vi "Example Websockets Client-Server.vi"() -> ()   [LabVIEW 2013]
uses:
  <vilib>/LabVIEW Open Source Project/Connection/Connection/Connection.lvclass
  MQTT_Websockets/Connection/WebsocketsConnection.lvclass
panel:
  out "server connected":bool
  out "client connected":bool
  out "Comm OK":bool
  out "value":dbl
  out "listener error":errorcluster
  out "client session error":errorcluster
  out "server session error":errorcluster
  out "Bytes":u8[](array[numeric]) format="%08b"
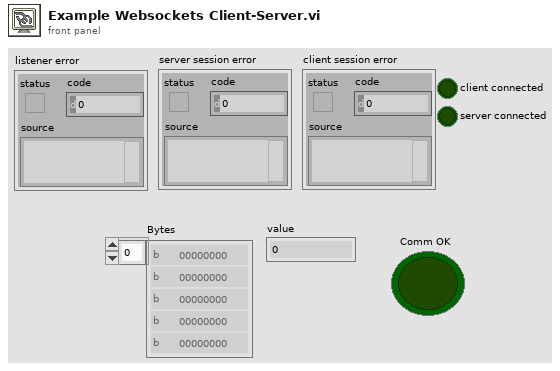
[diagram p1: front panel]
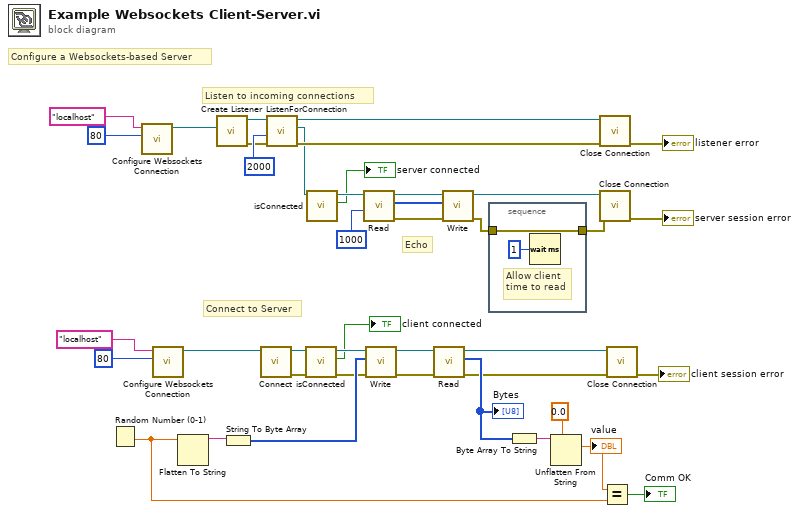
[diagram p0: block diagram]
diagram:
  # "Connect to Server"
  # "Echo"
  # "Listen to incoming connections"
  # "Configure a Websockets-based Server"
  n1 = Random Number (0-1)() -> (number: 0 to 1=w18:dbl)
  n2 = call "Configure Websockets Connection.vi"("remote port (80)"=u16 80, "address (localhost)"="localhost") -> ("WSConnection"=w14:refnum<class "WebsocketsConnection.lvclass">)  [unwired: 8 in, 1 out]
  n3 = call "Configure Websockets Connection.vi"("remote port (80)"=u16 80, "address (localhost)"="localhost") -> ("WSConnection"=w13:refnum<class "WebsocketsConnection.lvclass">)  [unwired: 8 in, 1 out]
  n4 = Flatten To String(anything=w18) -> (data string=w29:string)  [unwired: 3 in, 2 out]
  n5 = call <vilib>:"Create Listener.vi"("Connection Configuration"=w14) -> ("error out"=w38:errorcluster, "Listener"=w41:refnum<class "WebsocketsConnection.lvclass">)  [unwired: 9 in]
  n6 = String To Byte Array(string=w29) -> (unsigned byte array=w28:u8[])
  n7 = call <vilib>:"Connect.vi"("Connection in"=w13) -> ("error out"=w6:errorcluster, "Connection out"=w4:refnum<class "WebsocketsConnection.lvclass">)  [unwired: 9 in]
  n8 = call <vilib>:"ListenForConnection.vi"("error in (no error)"=w38, "timeout (2000 ms)"=2000 ("bytes to read (100)"), "Listener"=w41) -> ("error out"=w23:errorcluster, "Connection"=w8:refnum<class "Connection.lvclass">, "Listener out"=w39:refnum<class "WebsocketsConnection.lvclass">)  [unwired: 5 in, 1 out]
  n9 = call <vilib>:"isConnected.vi"("error in (no error)"=w6, "Connection in"=w4) -> ("error out"=w5:errorcluster, "connected"=→"client connected":bool, "Connection out"=w3:refnum<class "WebsocketsConnection.lvclass">)  [unwired: 7 in]
  n10 = call <vilib>:"isConnected.vi"("Connection in"=w8) -> ("connected"=→"server connected":bool, "Connection out"=w7:refnum<class "Connection.lvclass">)  [unwired: 8 in, 1 out]
  n11 = call <vilib>:"Read.vi"("timeout (2000 ms)"=1000 ("bytes to read (100)"), "TCPConnection in"=w7) -> ("error out"=w33:errorcluster, "Bytes"=w35:u8[], "TCPConnection out"=w36:refnum<class "Connection.lvclass">)  [unwired: 5 in, 2 out]
  n12 = call <vilib>:"Write.vi"("error in (no error)"=w5, "Bytes"=w28, "Connection in"=w3) -> ("error out"=w32:errorcluster, "Connection"=w34:refnum<class "WebsocketsConnection.lvclass">)  [unwired: 7 in]
  n13 = call <vilib>:"Read.vi"("error in (no error)"=w32, "TCPConnection in"=w34) -> ("error out"=w21:errorcluster, "Bytes"=w27:u8[], "TCPConnection out"=w20:refnum<class "WebsocketsConnection.lvclass">)  [unwired: 5 in, 2 out]
  "Bytes" <- w27
  n14 = call <vilib>:"Write.vi"("error in (no error)"=w33, "Bytes"=w35, "Connection in"=w36) -> ("error out"=w16:errorcluster, "Connection"=w30:refnum<class "Connection.lvclass">)  [unwired: 7 in]
  n15 = stacked-sequence {
    tunnel: w16 -> [w42]
    tunnel: [w42] -> w15
    frame #0 {
      # "Allow client\ntime to read"
      n16 = Wait (ms)(milliseconds to wait=u32 1) -> ()  [unwired: 1 out]
    }
  }
  n17 = Byte Array To String(unsigned byte array=w27) -> (string=w26:string)
  n18 = Unflatten From String(type=0.0, binary string=w26) -> (value=w19:dbl)  [unwired: 3 in, 2 out]
  "value" <- w19
  n19 = call <vilib>:"Close Connection.vi"("error in (no error)"=w23, "Connection in"=w39) -> ("error out"=→"listener error":errorcluster)  [unwired: 8 in, 1 out]
  n20 = call <vilib>:"Close Connection.vi"("error in (no error)"=w15, "Connection in"=w30) -> ("error out"=→"server session error":errorcluster)  [unwired: 8 in, 1 out]
  n21 = Equal?(x=w19, y=w18) -> (x = y?=→"Comm OK":bool)
  n22 = call <vilib>:"Close Connection.vi"("error in (no error)"=w21, "Connection in"=w20) -> ("error out"=→"client session error":errorcluster)  [unwired: 8 in, 1 out]
